vi "Load Help File.vi"(8 "error in (no error)":errorcluster, 9 "HTML File to Load":string, 11 "SHDocVw.IWebBrowser2":refnum<k7>(container)) -> (0 "error out":errorcluster)   [LabVIEW 2020, in "Instrument Addon System Explorer.lvlib"]
uses:
  Instrument Addon System Explorer.lvlib
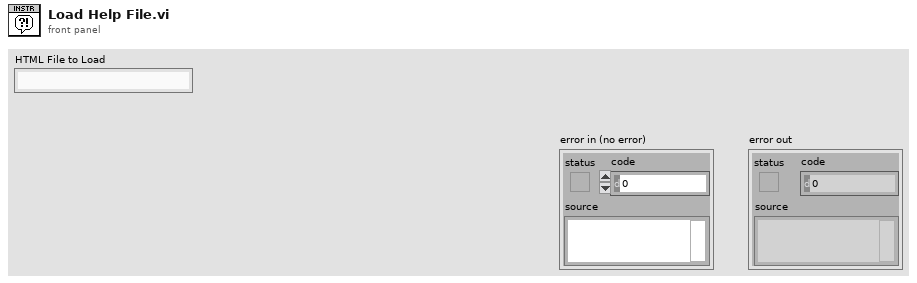
[diagram p1: front panel]
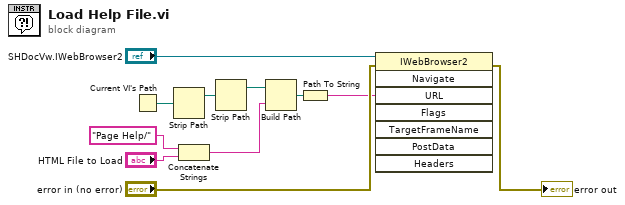
[diagram p0: block diagram]
diagram:
  n1 = Current VI's Path() -> (path=w11:path)
  n2 = Strip Path(path=w11) -> (stripped path=w10:path)  [unwired: 1 out]
  n3 = Concatenate Strings("Page Help/" ("Main CHM File"), "HTML File to Load") -> (w1:string)
  n4 = Strip Path(path=w10) -> (stripped path=w9:path)  [unwired: 1 out]
  n5 = Build Path(base path=w9, name or relative path=w1) -> (appended path=w8:path)
  n6 = Path To String(path=w8) -> (string=w4:string)
  n7 = invoke class="IWebBrowser2" method="Navigate"(reference="SHDocVw.IWebBrowser2", error in="error in (no error)", "URL"=w4) -> (error out=→"error out":errorcluster)  [unwired: 5 in, 7 out]
